vi "Table, Get Cell Value.vi"(8 "error in":errorcluster, 9 "column (0)":u32, 10 "row (0)":u32, 11 "Tbl Refnum":refnum<vi>) -> (0 "error out":errorcluster, 2 "cell value":string, 3 "Tbl Refnum out":refnum<vi>)   [LabVIEW 2020]
doc: "Gets a single table cell string value."
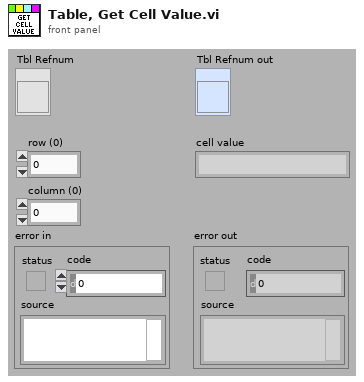
[diagram p1: front panel]
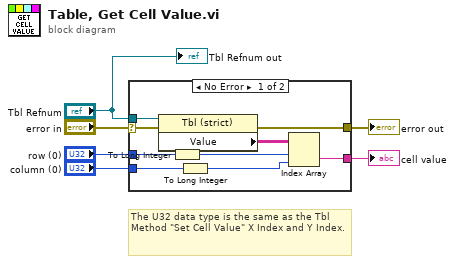
[diagram p0: block diagram]
diagram:
  # "The U32 data type is the same as the Tbl Method \"Set Cell Value\" X Index and Y Index."
  n1 = case shown="No Error" "error in" {
    selector: "error in" -> [w13 w16]
    tunnel: "Tbl Refnum" -> [w15 _]
    tunnel: [w14 w16] -> w5
    tunnel: "row (0)" -> [w11 _]
    tunnel: "column (0)" -> [w10 _]
    tunnel: [w9 _] -> w1
    frame No Error {
      n2 = property class="Tbl (strict)"(reference=w15, error in=w13) -> (error out=w14:errorcluster, "Value"=w12:string[][])  [unwired: 1 out]
      n3 = To Long Integer(number=w11) -> (32bit integer=w8:i32)
      n4 = To Long Integer(number=w10) -> (32bit integer=w7:i32)
      n5 = Index Array(array=w12, index (row)=w8, index (col)=w7) -> (element=w9:string)
    }
    frame Error {
    }
  }
  "error out" <- w5
  "cell value" <- w1
  "Tbl Refnum out" <- "Tbl Refnum"
